vi "TCPIPServidorTeste.vi"() -> ()   [LabVIEW 2018]
uses:
  CCDCamera/CCDCamera.lvclass
  CCDCamera/CCDCamera.lvclass/CCDCamera.ctl
panel:
  in  "CCDCamera in":refnum<class "CCDCamera.lvclass">
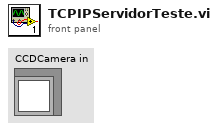
[diagram p1: front panel]
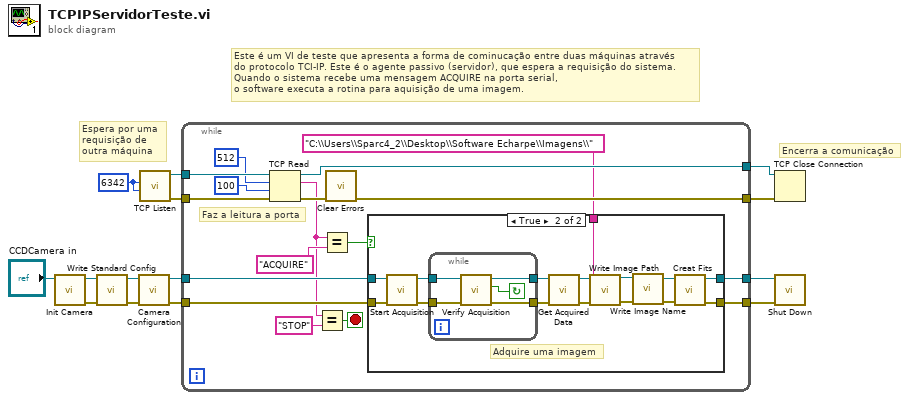
[diagram p0: block diagram]
diagram:
  w2 = u16 6342 ("port")
  # "Encerra a comunicação"
  # "Este é um VI de teste que apresenta a forma de cominucação entre duas máquinas através\ndo protocolo TCI-IP. Este é o agente passivo (servidor), que espera a requisição do sistema.\nQuando o sistema recebe uma mensagem ACQUIRE na porta serial,\no software executa a rotina para aquisição de uma imagem."
  # "Espera por uma \nrequisição de \noutra máquina"
  n1 = call "Init Camera.vi"("CCDCamera in"="CCDCamera in") -> ("error out"=w13:errorcluster, "CCDCamera out"=w14:refnum<class "CCDCamera.lvclass">)  [unwired: 9 in]
  n2 = call "Write Standard Config.vi"("error in (no error)"=w13, "CCDCamera in"=w14) -> ("error out"=w12:errorcluster, "CCDCamera out"=w11:refnum<class "CCDCamera.lvclass">)  [unwired: 8 in]
  n3 = call "Camera Configuration.vi"("error in (no error)"=w12, "CCDCamera in"=w11) -> ("error out"=w8:errorcluster, "CCDCamera out"=w10:refnum<class "CCDCamera.lvclass">)  [unwired: 8 in]
  n4 = call <vilib>:"TCP Listen.vi"("timeout ms (wait forever: -1)"=w2, "port"=w2) -> ("error out"=w7:errorcluster, "connection ID"=w6:refnum<k5>)  [unwired: 5 in, 3 out]
  n5 = while {
    tunnel: w10 -> [w31]
    tunnel: [w30] -> w9
    tunnel: [w29] -> w1
    tunnel: w8 -> [w28]
    tunnel: w7 -> [w27]
    tunnel: w6 -> [w26]
    tunnel: [w20] -> w5
    tunnel: [w19] -> w4
    stop <- w16 stop-if-true
    # "Faz a leitura a porta"
    n6 = TCP Read(connection ID=w26, bytes to read=512, error in (no error)=w27, 9:100 ("timeout ms (25000)")) -> (connection ID out=w19:refnum<k5>, data out=w15:string, error out=w21:errorcluster)  [unwired: 1 in]
    n7 = Equal?(x=w15, y="STOP") -> (x = y?=w16:bool)
    n8 = Equal?(x=w15, y="ACQUIRE") -> (x = y?=w22:bool)
    n9 = call <vilib>:"Clear Errors.vi"("error in (no error)"=w21) -> ("error out"=w20:errorcluster)  [unwired: 5 in, 1 out]
    n10 = case shown="True" w22 {
      tunnel: w31 -> [w33 w44]
      tunnel: [w32 w43] -> w30
      tunnel: [w33 w42] -> w29
      tunnel: w28 -> [w32 w41]
      tunnel: "C:\\Users\\Sparc4_2\\Desktop\\Software Echarpe\\Imagens\\" ("Image Path") -> [_ w40]
      frame False {
      }
      frame True {
        # "Adquire uma imagem"
        n11 = call "Start Acquisition.vi"("error in (no error)"=w41, "CCDCamera in"=w44) -> ("error out"=w48:errorcluster, "CCDCamera out"=w47:refnum<class "CCDCamera.lvclass">)  [unwired: 8 in]
        n12 = while {
          tunnel: w48 -> [w53]
          tunnel: [w52] -> w46
          tunnel: [w51] -> w45
          tunnel: w47 -> [w50]
          stop <- w49 continue-if-true
          n13 = call "Verify Acquisition.vi"("error in (no error)"=w53, "CCDCamera in"=w50) -> ("error out"=w52:errorcluster, "Acquiring"=w49:bool, "CCDCamera out"=w51:refnum<class "CCDCamera.lvclass">)  [unwired: 7 in]
        }
        n14 = call "Get Acquired Data.vi"("error in (no error)"=w46, "CCDCamera in"=w45) -> ("error out"=w39:errorcluster, "CCDCamera out"=w38:refnum<class "CCDCamera.lvclass">)  [unwired: 8 in]
        n15 = call "Write Image Path.vi"("error in (no error)"=w39, "Image Path"=w40, "CCDCamera in"=w38) -> ("error out"=w37:errorcluster, "CCDCamera out"=w34:refnum<class "CCDCamera.lvclass">)  [unwired: 7 in]
        n16 = call "Write Image Name.vi"("error in (no error)"=w37, "CCDCamera in"=w34) -> ("error out"=w36:errorcluster, "CCDCamera out"=w35:refnum<class "CCDCamera.lvclass">)  [unwired: 8 in]
        n17 = call "Creat Fits.vi"("error in (no error)"=w36, "CCDCamera in"=w35) -> ("error out"=w43:errorcluster, "CCDCamera out"=w42:refnum<class "CCDCamera.lvclass">)  [unwired: 8 in]
      }
    }
  }
  n18 = TCP Close Connection(connection ID=w4, error in (no error)=w5) -> ()  [unwired: 1 in, 2 out]
  n19 = call "Shut Down.vi"("error in (no error)"=w9, "CCDCamera in"=w1) -> ()  [unwired: 8 in, 2 out]
